vi "data_Create Notifiers.vi"(8 "error in":errorcluster) -> (0 "error out":errorcluster, 3 "output cluster":T1)   [LabVIEW 2017]
uses:
  data_Notifiers.ctl
  measurement_result/MeasurementResult.lvclass
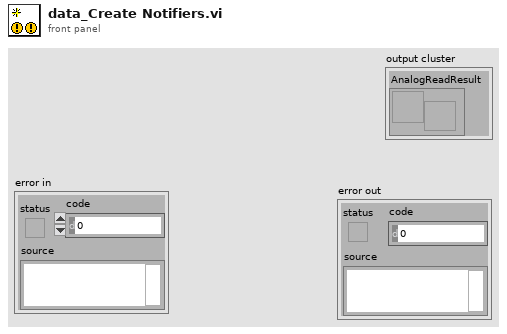
[diagram p1: front panel]
types:
  T1 = typedef "data_Notifiers.ctl" = cluster{"AnalogReadResult":refnum<notifier>}
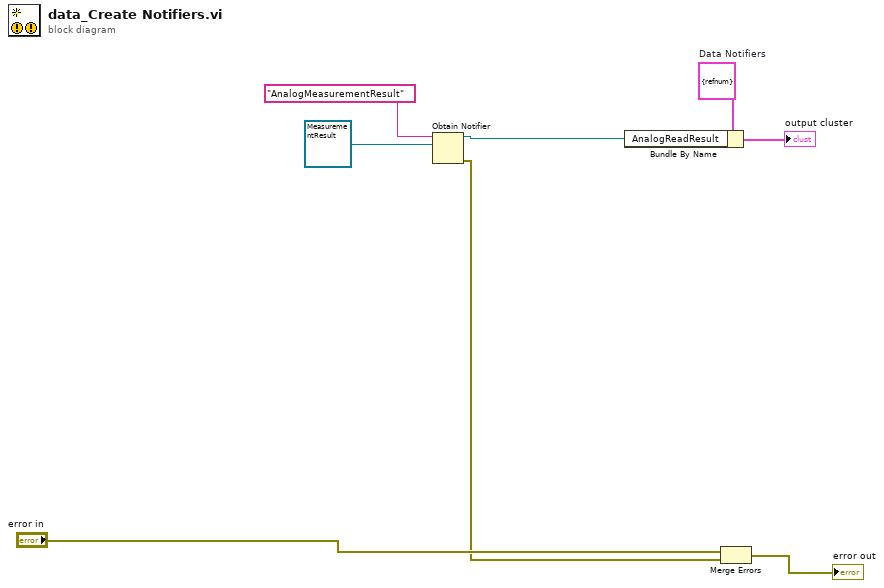
[diagram p0: block diagram]
diagram:
  w4 = T1 {"AnalogReadResult"=refnum}  # Data Notifiers
  n1 = Obtain Notifier(name (unnamed)="AnalogMeasurementResult", notification data type=refnum<class "MeasurementResult.lvclass"> refnum ("MeasurementResult.lvclass")) -> (notifier out=w3:refnum<notifier>, error out=w1:errorcluster)  [unwired: 2 in, 1 out]
  n2 = Bundle By Name(cluster=w4, "AnalogReadResult"=w3) -> (→"output cluster":T1)
  n3 = Merge Errors("error in", w1) -> (→"error out":errorcluster)
